vi "Py - NametoZ.vi"(7 "python in":refnum<k35>, 8 "error in":errorcluster, 11 "Name Element":string) -> (0 "error out":errorcluster, 3 "Z":i32, 5 "python out":refnum<k35>)   [LabVIEW 2023]
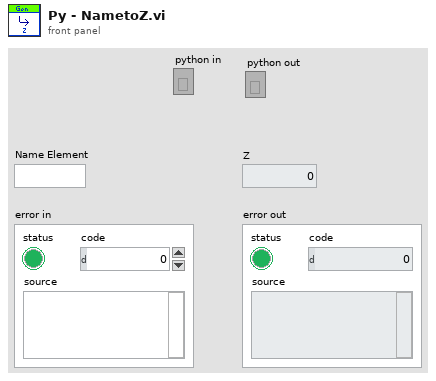
[diagram p1: front panel]
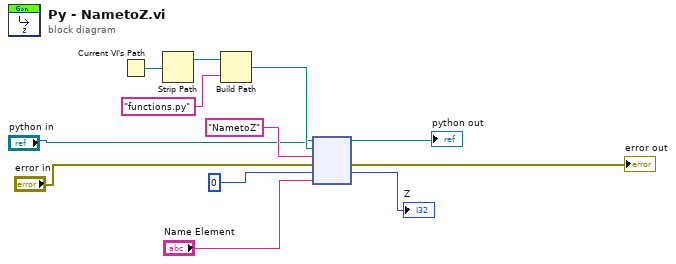
[diagram p0: block diagram]
diagram:
  n1 = Current VI's Path() -> (path=w11:path)
  n2 = Strip Path(path=w11) -> (stripped path=w10:path)  [unwired: 1 out]
  n3 = Build Path(base path=w10, name or relative path="functions.py") -> (appended path=w7:path)
  n4 = node("python in", w7, "NametoZ", "error in", 0, "Name Element") -> (→"python out":refnum<k35>, →"error out":errorcluster, →"Z":i32)  [unwired: 1 in, 2 out]
